vi "MAIN_old.vi"() -> ()   [LabVIEW 2011]
uses:
  <vilib>/userDefined/High Color/IMAQdx.ctl
  <vilib>/vision/driver/NI_Vision_Acquisition_Software.lvlib
panel:
  out "error out 3":errorcluster
  out "error out 2":errorcluster
  out "error out":errorcluster
  out "Image":T1(plugin-control)
  in  "Focused":bool
  out "Ph2 2":dbl
  out "Ph1 2":dbl
  out "[0 255]":dbl
  out "[0 255]":dbl
  in  "Semi2":bool caption="Boolean"
  in  "Semi":bool caption="Boolean"
  out "path":path
  in  "Phase correction 2":bool
  in  "Phase correction":bool caption="Amplitude correction"
  in  "M4":bool
  in  "M4":bool caption="Amplitude correction"
  in  "Hologram:":dbl=1.0
  in  "Hologram:":dbl=1.0
  out "String 2":string
  out "String":string
  out "Ph2":dbl
  in  "Phase:":dbl(slide) scale=0.0..360.0
  out "T2":dbl=100.0
  in  "Tranmitance:":dbl(slide)=100.0 scale=0.0..255.0
  out "Ph1":dbl
  in  "Phase:":dbl(slide) scale=0.0..360.0
  out "T1":dbl=100.0
  in  "Tranmitance:":dbl(slide)=100.0 scale=0.0..255.0
  in  "Parada Total":bool
  in  "Radio Buttons 2":T2(radio)=enum."Radio Selection 6"
  in  "Radio Buttons":T2(radio)=enum."Radio Selection 6"
  in  "Save":bool
  in  "Load Y":bool
  out "selected path 2":path
  in  "Load X":bool
  out "selected path":path
  out "Y position 2":dbl
  in  "Y position 2":dbl(slide)=3.9208633093525176 scale=0.0..10.0
  in  "Fine:":dbl(slide)=5.899280575539568 scale=0.0..10.0
  out "X 2":dbl
  in  "Fine:":dbl(slide)=2.2049689440993787 scale=0.0..10.0
  in  "X position 2":dbl(slide)=1.6770186335403727 scale=0.0..10.0
  out "Y position 1":dbl
  out "X position":dbl
  in  "Fine:":dbl(slide)=0.7636363636363636 scale=0.0..10.0
  in  "Fine:":dbl(slide)=5.590062111801243 scale=0.0..10.0
  in  "X position 1":dbl(slide)=8.409785932721713 scale=0.0..10.0
  in  "Y position":dbl(slide)=2.9454545454545453 scale=0.0..10.0
  out "CGH_x >>":T1(plugin-control)
  out "<< CGH_y":T1(plugin-control)
  # "Arbitrary value settings:"
  # "For gray levels ->"
  # "%"
  # "º"
  # "\\pi rad"
  # "Paraxial"
  # "Arbitrary value settings:"
  # "For gray levels ->"
  # "%"
  # "º"
  # "\\pi rad"
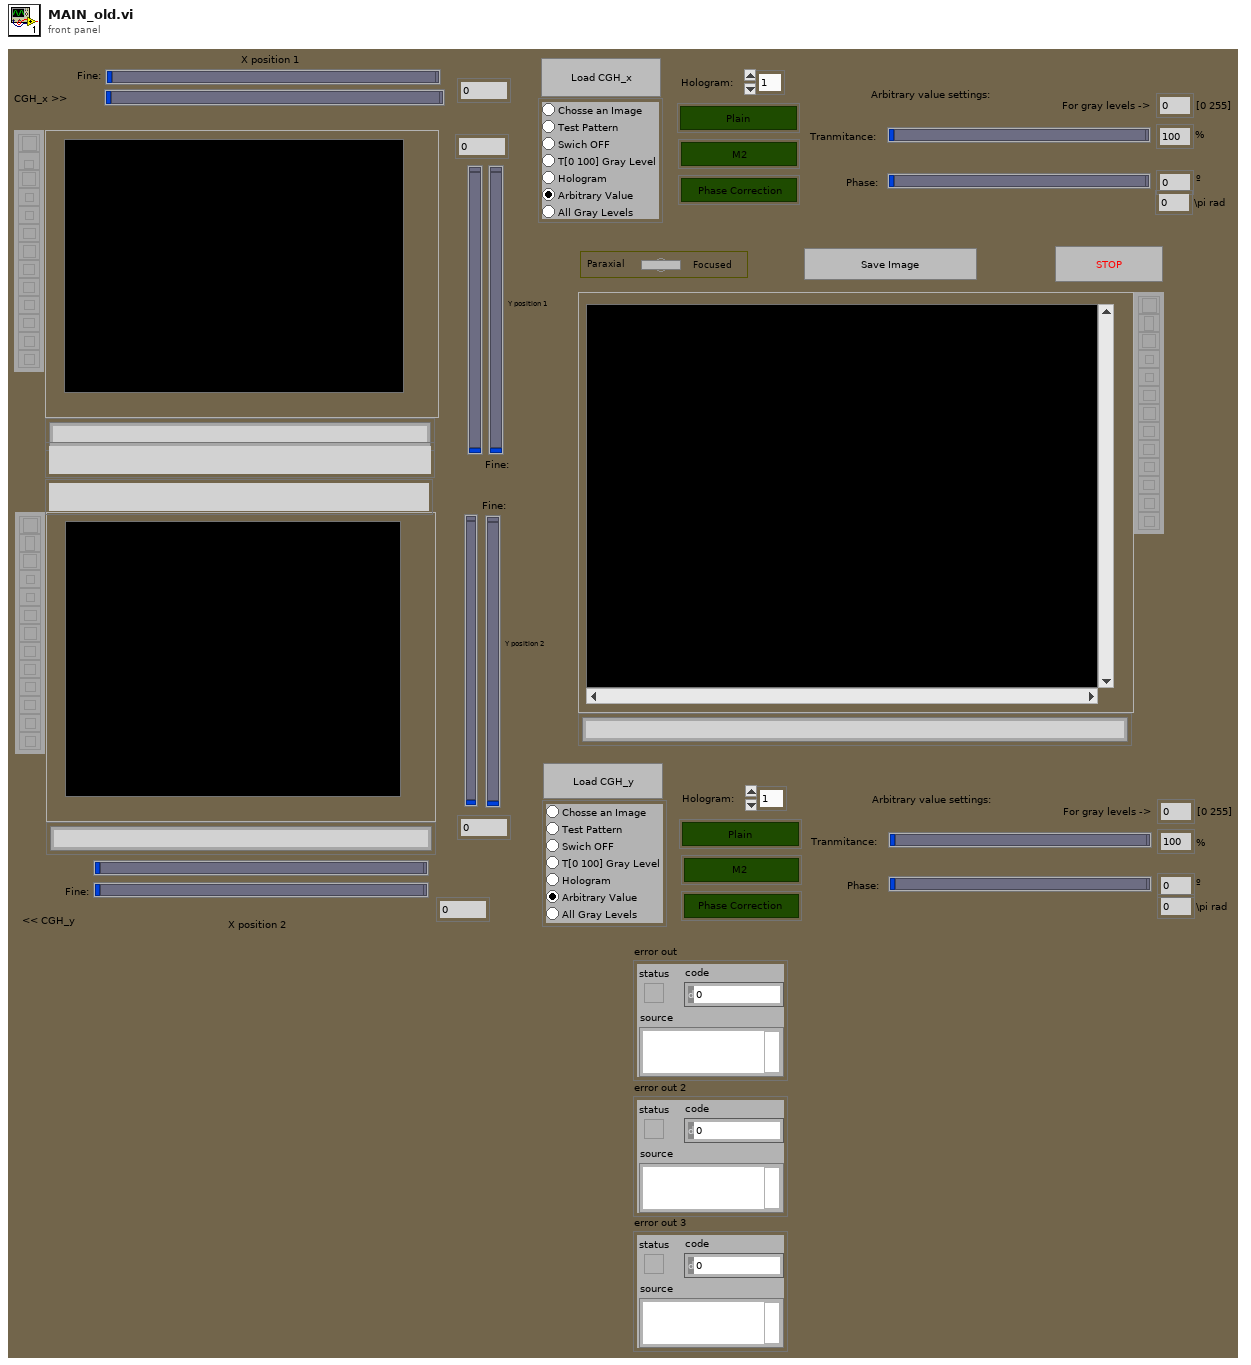
[diagram p1: front panel]
types:
  T1 = typedef "IMAQ Image.ctl" = refnum<image>
  T2 = enum32{"Radio Selection 1", "Radio Selection 2", "Radio Selection 3", "Radio Selection 4", "Radio Selection 5", "Radio Selection 6", "Radio Selection 7"}
  T3 = typedef "IMAQdx.ctl" = refnum<k21>
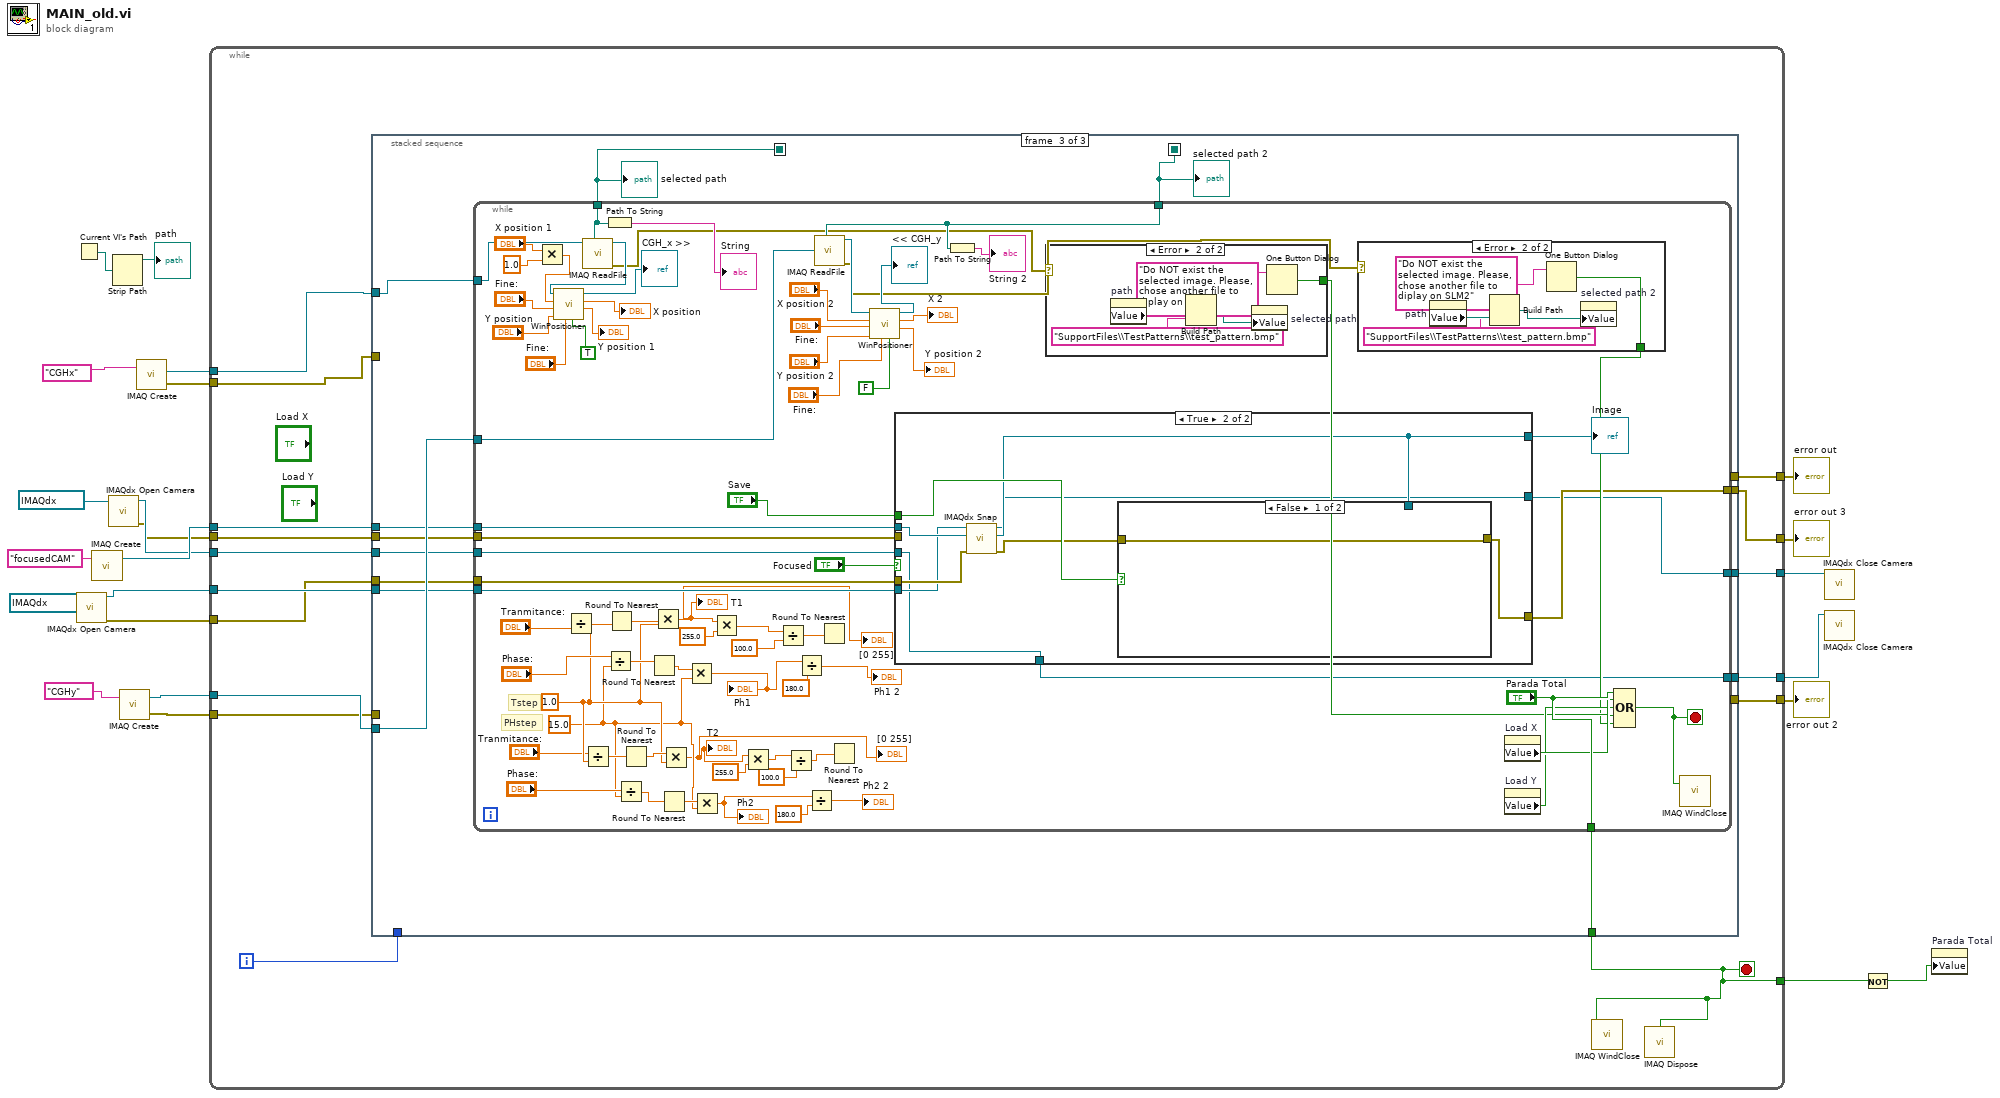
[diagram p0: block diagram]
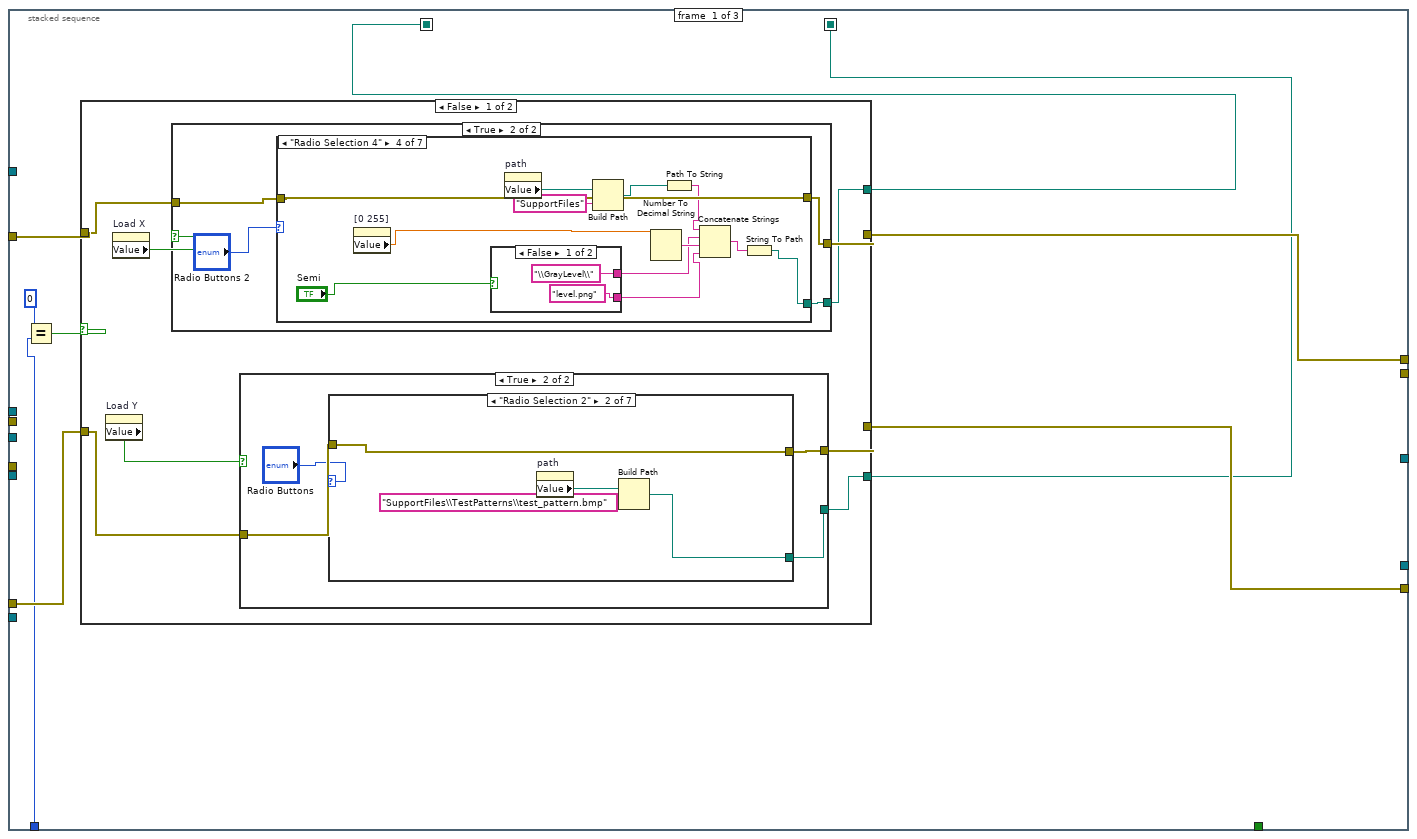
[diagram p2: hidden frame]
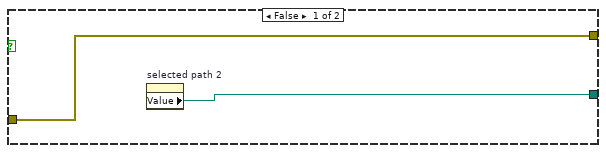
[diagram p3: hidden frame]
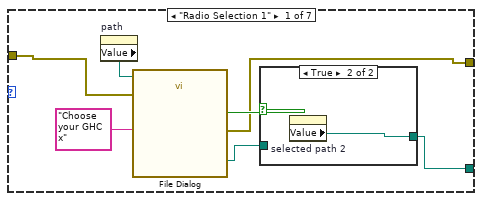
[diagram p4: hidden frame]
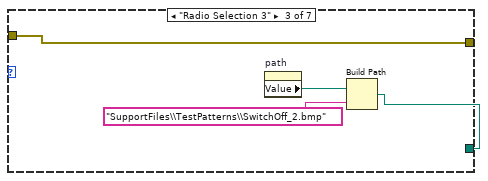
[diagram p6: hidden frame]
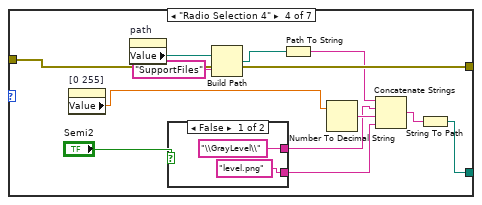
[diagram p7: hidden frame]
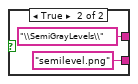
[diagram p8: hidden frame]
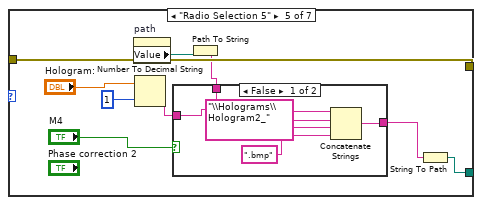
[diagram p9: hidden frame]
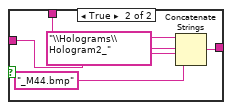
[diagram p10: hidden frame]
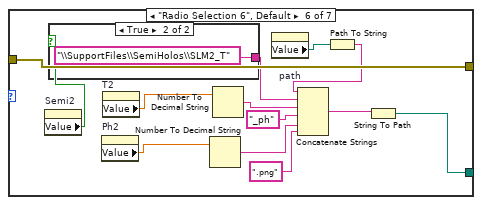
[diagram p11: hidden frame]
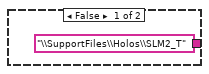
[diagram p12: hidden frame]
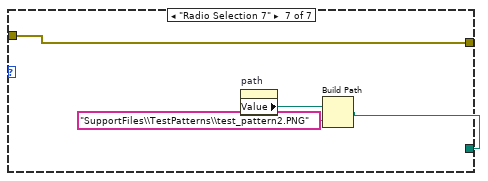
[diagram p13: hidden frame]
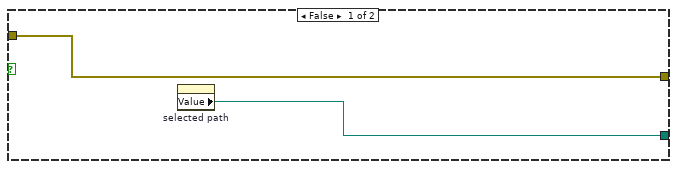
[diagram p14: hidden frame]
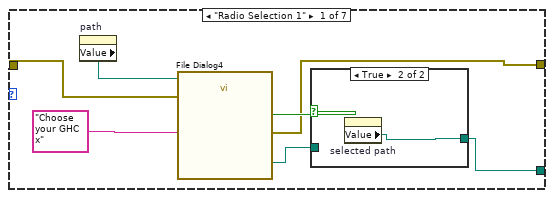
[diagram p15: hidden frame]
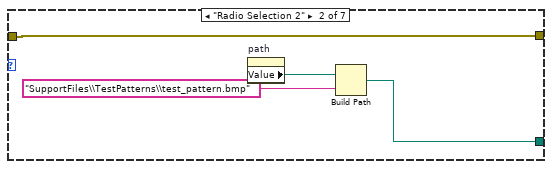
[diagram p17: hidden frame]
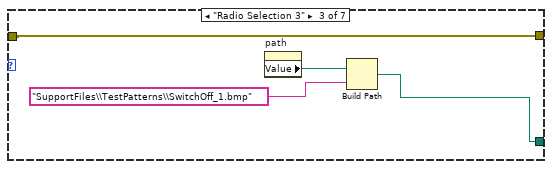
[diagram p18: hidden frame]
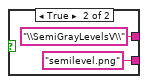
[diagram p19: hidden frame]
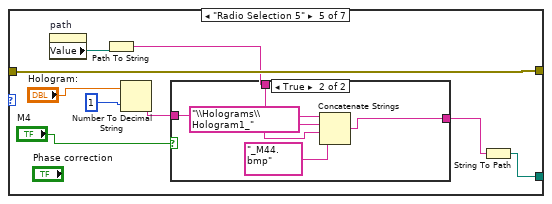
[diagram p20: hidden frame]
diagram:
  n1 = Current VI's Path() -> (path=w16:path)
  n2 = call <vilib>:"IMAQdx Open Camera.vi"("Session In"=T3 "Focused") -> ("error out"=w6:errorcluster, "Session Out"=w7:T3)  [unwired: 9 in]
  n3 = call "IMAQ Create"("Image Name"="focusedCAM") -> ("New Image"=w12:T1)  [unwired: 4 in, 1 out]
  n4 = call <vilib>:"IMAQdx Open Camera.vi"("Session In"=T3 "Paraxial") -> ("error out"=w9:errorcluster, "Session Out"=w10:T3)  [unwired: 9 in]
  n5 = Strip Path(path=w16) -> (stripped path=→"path":path)  [unwired: 1 out]
  n6 = call "IMAQ Create"("Image Name"="CGHy") -> ("New Image"=w20:T1, "error out"=w18:errorcluster)  [unwired: 4 in]
  n7 = call "IMAQ Create"("Image Name"="CGHx") -> ("New Image"=w21:T1, "error out"=w17:errorcluster)  [unwired: 4 in]
  n8 = while {
    tunnel: w21 -> [w39]
    tunnel: w20 -> [w38]
    tunnel: w18 -> [w37]
    tunnel: [w36] -> w4
    tunnel: w17 -> [w35]
    tunnel: [w34] -> w5
    tunnel: [w32] -> w14
    tunnel: w12 -> [w31]
    tunnel: w10 -> [w30]
    tunnel: w9 -> [w29]
    tunnel: w7 -> [w28]
    tunnel: w6 -> [w27]
    tunnel: [w26] -> w3
    tunnel: [w25] -> w2
    tunnel: [w24] -> w1
    i -> [w33]
    stop <- w32 stop-if-true
    n9 = stacked-sequence {
      seq-local: [w40 _ _] -> [_ _ w226]
      seq-local: [w41 _ _] -> [_ _ w225]
      tunnel: w39 -> [_ _ w227]
      tunnel: w38 -> [_ _ w228]
      tunnel: [_ _ w229] -> w32
      tunnel: w37 -> [w48 _ _]
      tunnel: [w47 _ _] -> w36
      tunnel: w35 -> [w46 _ _]
      tunnel: [w45 _ _] -> w34
      tunnel: w33 -> [w44 _ _]
      tunnel: [_ _ w224] -> w26
      tunnel: w31 -> [_ _ w223]
      tunnel: w30 -> [_ _ w222]
      tunnel: w29 -> [_ _ w221]
      tunnel: w28 -> [_ _ w220]
      tunnel: w27 -> [_ _ w219]
      tunnel: [_ _ w218] -> w25
      tunnel: [_ _ w217] -> w24
      frame #0 {
        n10 = Equal?(x=0, y=w44) -> (x = y?=w42:bool)
        n11 = case shown="False" w42 {
          tunnel: [w51 w211] -> w40
          tunnel: [w56 w211] -> w41
          tunnel: w48 -> [w50 w214]
          tunnel: [w53 w214] -> w47
          tunnel: w46 -> [w49 w215]
          tunnel: [w52 w215] -> w45
          frame False {
            n12 = property on="Load Y" class="Bool (strict)"() -> ("Value"=w55:bool)  [unwired: 2 in, 2 out]
            n13 = property on="Load X" class="Bool (strict)"() -> ("Value"=w54:bool)  [unwired: 2 in, 2 out]
            n14 = case shown="True" w54 {
              tunnel: [w135 w138] -> w51
              tunnel: w49 -> [w134 w139]
              tunnel: [w134 w137] -> w52
              frame False {
                n15 = property on="selected path" class="Path"() -> ("Value"=w135:path)  [unwired: 2 in, 2 out]
              }
              frame True {
                n16 = case shown="\"Radio Selection 4\"" "Radio Buttons 2" {
                  tunnel: w139 -> [w142 w152 w156 w168 w181 w204 w210]
                  tunnel: [w141 w149 w153 w165 w179 w198 w207] -> w138
                  tunnel: [w143 w152 w156 w168 w181 w204 w210] -> w137
                  frame "Radio Selection 1" {
                    n17 = property on="path" class="Path"() -> ("Value"=w140:path)  [unwired: 2 in, 2 out]
                    n18 = call "File Dialog4"("start path"=w140, "prompt"="Choose your GHC x", "error in"=w142) -> ("selected path"=w145:path, "cancelled"=w144:bool, "error out"=w143:errorcluster)  [unwired: 9 in, 1 out]
                    n19 = case shown="True" w144 {
                      tunnel: [w147 w148] -> w141
                      tunnel: w145 -> [w147 _]
                      frame False {
                      }
                      frame True {
                        n20 = property on="selected path" class="Path"() -> ("Value"=w148:path)  [unwired: 2 in, 2 out]
                      }
                    }
                  }
                  frame "Radio Selection 2" {
                    n21 = property on="path" class="Path"() -> ("Value"=w151:path)  [unwired: 2 in, 2 out]
                    n22 = Build Path(base path=w151, name or relative path="SupportFiles\\TestPatterns\\test_pattern.bmp") -> (appended path=w149:path)
                  }
                  frame "Radio Selection 3" {
                    n23 = property on="path" class="Path"() -> ("Value"=w155:path)  [unwired: 2 in, 2 out]
                    n24 = Build Path(base path=w155, name or relative path="SupportFiles\\TestPatterns\\SwitchOff_1.bmp") -> (appended path=w153:path)
                  }
                  frame "Radio Selection 4" {
                    n25 = property on="[0 255]" class="DigNum (strict)"() -> ("Value"=w157:dbl)  [unwired: 2 in, 2 out]
                    n26 = case shown="False" "Semi" {
                      tunnel: ["\\GrayLevel\\" ("name or relative path") "\\SemiGrayLevelsV\\" ("name or relative path")] -> w159
                      tunnel: ["level.png" ("string") "semilevel.png" ("string")] -> w158
                      frame False {
                      }
                      frame True {
                      }
                    }
                    n27 = property on="path" class="Path"() -> ("Value"=w164:path)  [unwired: 2 in, 2 out]
                    n28 = Build Path(base path=w164, name or relative path="SupportFiles") -> (appended path=w162:path)
                    n29 = Number To Decimal String(number=w157) -> (decimal integer string=w167:string)  [unwired: 1 in]
                    n30 = Path To String(path=w162) -> (string=w161:string)
                    n31 = Concatenate Strings(w161, w159, w167, w158) -> (w166:string)
                    n32 = String To Path(string=w166) -> (path=w165:path)
                  }
                  frame "Radio Selection 5" {
                    n33 = property on="path" class="Path"() -> ("Value"=w174:path)  [unwired: 2 in, 2 out]
                    n34 = Path To String(path=w174) -> (string=w173:string)
                    n35 = Number To Decimal String(number="Hologram:", width (-)=i16 1) -> (decimal integer string=w177:string)
                    n36 = case shown="True" "M4" {
                      tunnel: [w185 w189] -> w180
                      tunnel: w177 -> [w184 w188]
                      tunnel: w173 -> [w183 w187]
                      frame False {
                        n37 = Concatenate Strings(w183, "\\Holograms\\Hologram1_" ("string"), w184, ".bmp" ("string")) -> (w185:string)
                      }
                      frame True {
                        n38 = Concatenate Strings(w187, "\\Holograms\\Hologram1_" ("string"), w188, "_M44.bmp" ("string")) -> (w189:string)
                      }
                    }
                    n39 = String To Path(string=w180) -> (path=w179:path)
                  }
                  frame "Radio Selection 6", Default {
                    n40 = property on="Semi" class="Bool (strict)"() -> ("Value"=w192:bool)  [unwired: 2 in, 2 out]
                    n41 = case shown="True" w192 {
                      tunnel: ["\\SupportFiles\\Holos\\SLM1_T" ("name or relative path") "\\SupportFiles\\SemiHolos\\SLM1_T" ("name or relative path")] -> w193
                      frame False {
                      }
                      frame True {
                      }
                    }
                    n42 = property on="T1" class="DigNum (strict)"() -> ("Value"=w197:dbl)  [unwired: 2 in, 2 out]
                    n43 = property on="Ph1" class="DigNum (strict)"() -> ("Value"=w196:dbl)  [unwired: 2 in, 2 out]
                    n44 = property on="path" class="Path"() -> ("Value"=w195:path)  [unwired: 2 in, 2 out]
                    n45 = Number To Decimal String(number=w196) -> (decimal integer string=w202:string)  [unwired: 1 in]
                    n46 = Number To Decimal String(number=w197) -> (decimal integer string=w203:string)  [unwired: 1 in]
                    n47 = Path To String(path=w195) -> (string=w194:string)
                    n48 = Concatenate Strings(w194, w193, w203, "_ph" ("Master Thesis (folder)"), w202, ".png" ("Master Thesis (folder)")) -> (w199:string)
                    n49 = String To Path(string=w199) -> (path=w198:path)
                  }
                  frame "Radio Selection 7" {
                    n50 = property on="path" class="Path"() -> ("Value"=w209:path)  [unwired: 2 in, 2 out]
                    n51 = Build Path(base path=w209, name or relative path="SupportFiles\\TestPatterns\\test_pattern2V.PNG") -> (appended path=w207:path)
                  }
                }
              }
            }
            n52 = case shown="True" w55 {
              tunnel: [w58 w61] -> w56
              tunnel: w50 -> [w57 w62]
              tunnel: [w57 w59] -> w53
              frame False {
                n53 = property on="selected path 2" class="Path"() -> ("Value"=w58:path)  [unwired: 2 in, 2 out]
              }
              frame True {
                n54 = case shown="\"Radio Selection 2\"" "Radio Buttons" {
                  tunnel: w62 -> [w65 w75 w79 w91 w104 w127 w133]
                  tunnel: [w64 w72 w76 w88 w102 w121 w130] -> w61
                  tunnel: [w66 w75 w79 w91 w104 w127 w133] -> w59
                  frame "Radio Selection 1" {
                    n55 = property on="path" class="Path"() -> ("Value"=w63:path)  [unwired: 2 in, 2 out]
                    n56 = call "File Dialog"("start path"=w63, "prompt"="Choose your GHC x", "error in"=w65) -> ("selected path"=w68:path, "cancelled"=w67:bool, "error out"=w66:errorcluster)  [unwired: 9 in, 1 out]
                    n57 = case shown="True" w67 {
                      tunnel: [w70 w71] -> w64
                      tunnel: w68 -> [w70 _]
                      frame False {
                      }
                      frame True {
                        n58 = property on="selected path 2" class="Path"() -> ("Value"=w71:path)  [unwired: 2 in, 2 out]
                      }
                    }
                  }
                  frame "Radio Selection 2" {
                    n59 = property on="path" class="Path"() -> ("Value"=w74:path)  [unwired: 2 in, 2 out]
                    n60 = Build Path(base path=w74, name or relative path="SupportFiles\\TestPatterns\\test_pattern.bmp") -> (appended path=w72:path)
                  }
                  frame "Radio Selection 3" {
                    n61 = property on="path" class="Path"() -> ("Value"=w78:path)  [unwired: 2 in, 2 out]
                    n62 = Build Path(base path=w78, name or relative path="SupportFiles\\TestPatterns\\SwitchOff_2.bmp") -> (appended path=w76:path)
                  }
                  frame "Radio Selection 4" {
                    n63 = property on="[0 255]" class="DigNum (strict)"() -> ("Value"=w80:dbl)  [unwired: 2 in, 2 out]
                    n64 = property on="path" class="Path"() -> ("Value"=w87:path)  [unwired: 2 in, 2 out]
                    n65 = case shown="False" "Semi2" {
                      tunnel: ["\\GrayLevel\\" ("name or relative path") "\\SemiGrayLevels\\" ("name or relative path")] -> w83
                      tunnel: ["level.png" ("string") "semilevel.png" ("string")] -> w82
                      frame False {
                      }
                      frame True {
                      }
                    }
                    n66 = Build Path(base path=w87, name or relative path="SupportFiles") -> (appended path=w85:path)
                    n67 = Path To String(path=w85) -> (string=w84:string)
                    n68 = Number To Decimal String(number=w80) -> (decimal integer string=w90:string)  [unwired: 1 in]
                    n69 = Concatenate Strings(w84, w83, w90, w82) -> (w89:string)
                    n70 = String To Path(string=w89) -> (path=w88:path)
                  }
                  frame "Radio Selection 5" {
                    n71 = property on="path" class="Path"() -> ("Value"=w97:path)  [unwired: 2 in, 2 out]
                    n72 = Number To Decimal String(number="Hologram:", width (-)=i16 1) -> (decimal integer string=w98:string)
                    n73 = Path To String(path=w97) -> (string=w96:string)
                    n74 = case shown="False" "M4" {
                      tunnel: w96 -> [w107 w114]
                      tunnel: [w105 w111] -> w103
                      tunnel: w98 -> [w108 w112]
                      frame False {
                        n75 = Concatenate Strings(w107, "\\Holograms\\Hologram2_" ("string"), w108, ".bmp" ("string")) -> (w105:string)
                      }
                      frame True {
                        n76 = Concatenate Strings(w114, "\\Holograms\\Hologram2_" ("string"), w112, "_M44.bmp" ("string")) -> (w111:string)
                      }
                    }
                    n77 = String To Path(string=w103) -> (path=w102:path)
                  }
                  frame "Radio Selection 6", Default {
                    n78 = property on="Semi2" class="Bool (strict)"() -> ("Value"=w118:bool)  [unwired: 2 in, 2 out]
                    n79 = case shown="True" w118 {
                      tunnel: ["\\SupportFiles\\Holos\\SLM2_T" ("name or relative path") "\\SupportFiles\\SemiHolos\\SLM2_T" ("name or relative path")] -> w115
                      frame False {
                      }
                      frame True {
                      }
                    }
                    n80 = property on="Ph2" class="DigNum (strict)"() -> ("Value"=w119:dbl)  [unwired: 2 in, 2 out]
                    n81 = property on="T2" class="DigNum (strict)"() -> ("Value"=w120:dbl)  [unwired: 2 in, 2 out]
                    n82 = Number To Decimal String(number=w119) -> (decimal integer string=w125:string)  [unwired: 1 in]
                    n83 = Number To Decimal String(number=w120) -> (decimal integer string=w126:string)  [unwired: 1 in]
                    n84 = property on="path" class="Path"() -> ("Value"=w117:path)  [unwired: 2 in, 2 out]
                    n85 = Path To String(path=w117) -> (string=w116:string)
                    n86 = Concatenate Strings(w116, w115, w126, "_ph" ("Master Thesis (folder)"), w125, ".png" ("Master Thesis (folder)")) -> (w122:string)
                    n87 = String To Path(string=w122) -> (path=w121:path)
                  }
                  frame "Radio Selection 7" {
                    n88 = property on="path" class="Path"() -> ("Value"=w132:path)  [unwired: 2 in, 2 out]
                    n89 = Build Path(base path=w132, name or relative path="SupportFiles\\TestPatterns\\test_pattern2.PNG") -> (appended path=w130:path)
                  }
                }
              }
            }
          }
          frame True {
            n90 = property on="path" class="Path"() -> ("Value"=w213:path)  [unwired: 2 in, 2 out]
            n91 = Build Path(base path=w213, name or relative path="SupportFiles\\TestPatterns\\test_pattern.bmp") -> (appended path=w211:path)
          }
        }
      }
      frame #1 {
        w216 = FALSE ("Load X")
        n92 = property on="Radio Selection 6" class="Bool (strict)" props=["Value"]() -> ()  [unwired: 2 in, 3 out]
        n93 = property on="Radio Selection 6" class="Bool (strict)" props=["Value"]() -> ()  [unwired: 2 in, 3 out]
        n94 = property on="Load X" class="Bool (strict)"("Value"=w216) -> ()  [unwired: 2 in, 2 out]
        n95 = property on="Load Y" class="Bool (strict)"("Value"=w216) -> ()  [unwired: 2 in, 2 out]
      }
      frame #2 {
        n96 = while {
          tunnel: ["Parada Total"] -> w229
          tunnel: w226 -> [w284]
          tunnel: w225 -> [w272]
          tunnel: w228 -> [w303]
          tunnel: w227 -> [w302]
          tunnel: [w243] -> w224
          tunnel: w223 -> [w239]
          tunnel: w222 -> [w238]
          tunnel: w221 -> [w237]
          tunnel: w220 -> [w236]
          tunnel: w219 -> [w235]
          tunnel: [w234] -> w218
          tunnel: [w233] -> w217
          stop <- w249 stop-if-true
          w253 = 15.0 ("x")
          w262 = 1.0 ("x")
          # "PHstep"
          # "Tstep"
          n97 = Multiply(x="X position 1", y=1.0 ("x")) -> (x*y=w288:dbl)
          n98 = Divide(x="Tranmitance:", y=w262) -> (x/y=w270:dbl)
          n99 = call "IMAQ ReadFile"("File Path"=w284, "Image"=w302) -> ("error out"=w271:errorcluster, "Image Out"=w291:T1)  [unwired: 5 in, 3 out]
          n100 = call "WinPositioner.vi"("Image"=w291, "X position"=w288, "Fine X position"="Fine:", "Y position"="Y position", "Fine Y position"="Fine:", "Display?"=TRUE) -> ("CGH_x"=→"CGH_x >>":T1, "X position"=→"X position":dbl, "Y position"=→"Y position 1":dbl)  [unwired: 2 in]
          n101 = Divide(x="Tranmitance:", y=w262) -> (x/y=w264:dbl)
          n102 = Path To String(path=w284) -> (string=→"String":string)
          n103 = Divide(x="Phase:", y=w253) -> (x/y=w300:dbl)
          n104 = Round To Nearest(number=w270) -> (nearest integer value=w297:dbl)
          n105 = Divide(x="Phase:", y=w253) -> (x/y=w255:dbl)
          n106 = Round To Nearest(number=w264) -> (nearest integer value=w263:dbl)
          n107 = Round To Nearest(number=w300) -> (nearest integer value=w298:dbl)
          n108 = Multiply(x=w297, y=w262) -> (x*y=w230:dbl)
          "T1" <- w230
          "[0 255]" <- w230
          n109 = Round To Nearest(number=w255) -> (nearest integer value=w254:dbl)
          n110 = Multiply(x=w263, y=w262) -> (x*y=w231:dbl)
          "T2" <- w231
          "[0 255]" <- w231
          n111 = Multiply(x=w298, y=w253) -> (x*y=w265:dbl)
          "Ph1" <- w265
          n112 = Multiply(x=w254, y=w253) -> (x*y=w252:dbl)
          "Ph2" <- w252
          n113 = Multiply(x=w230, y=255.0) -> (x*y=w268:dbl)
          n114 = Multiply(x=w231, y=255.0) -> (x*y=w260:dbl)
          n115 = Divide(x=w268, y=100.0) -> (x/y=w266:dbl)
          n116 = Divide(x=w260, y=100.0) -> (x/y=w258:dbl)
          n117 = Divide(x=w265, y=180.0) -> (x/y=→"Ph1 2":dbl)
          n118 = Divide(x=w252, y=180.0) -> (x/y=→"Ph2 2":dbl)
          n119 = call "IMAQ ReadFile"("File Path"=w272, "Image"=w303) -> ("error out"=w240:errorcluster, "Image Out"=w274:T1)  [unwired: 5 in, 3 out]
          n120 = Round To Nearest(number=w266) -> ()  [unwired: 1 out]
          n121 = Round To Nearest(number=w258) -> ()  [unwired: 1 out]
          n122 = call "WinPositioner.vi"("Image"=w274, "X position"="X position 2", "Fine X position"="Fine:", "Y position"="Y position 2", "Fine Y position"="Fine:", "Display?"=FALSE) -> ("CGH_x"=→"<< CGH_y":T1, "X position"=→"X 2":dbl, "Y position"=→"Y position 2":dbl)  [unwired: 2 in]
          n123 = case shown="True" "Focused" {
            tunnel: "Save" -> [w312 w334]
            tunnel: [w313 w335] -> w243
            tunnel: [w311 w332] -> w241
            tunnel: w239 -> [w307 w333]
            tunnel: w238 -> [w310 w327]
            tunnel: w237 -> [w309 _]
            tunnel: w236 -> [w305 w329]
            tunnel: w235 -> [_ w331]
            tunnel: [w305 w328] -> w234
            tunnel: [w306 w327] -> w233
            frame False {
              n124 = call <vilib>:"IMAQdx Snap.vi"("error in"=w309, "Image In"=w307, "Session In"=w310) -> ("error out"=w308:errorcluster, "Image Out"=w311:T1, "Session Out"=w306:T3)  [unwired: 6 in]
              n125 = case shown="False" w312 {
                tunnel: [w314 w317] -> w313
                tunnel: w311 -> [_ w316]
                tunnel: w308 -> [w314 w315]
                frame False {
                }
                frame True {
                  n126 = property on="path" class="Path"() -> ("Value"=w325:path)  [unwired: 2 in, 2 out]
                  n127 = Build Path(base path=w325, name or relative path="Images") -> (appended path=w324:path)
                  n128 = call "File Dialog3"("start path"=w324, "prompt"="Save image", "button label"="Save", "error in"=w315, "pattern (all files)"=".png", "pattern label"="PNG") -> ("selected path"=w326:path, "error out"=w318:errorcluster)  [unwired: 6 in, 2 out]
                  n129 = call-poly "IMAQ Write File 2"("error in (no error)"=w318, "File Path"=w326, "Image"=w316) -> ("error out"=w317:errorcluster)  [unwired: 7 in, 1 out]
                }
              }
            }
            frame True {
              n130 = call <vilib>:"IMAQdx Snap.vi"("error in"=w331, "Image In"=w333, "Session In"=w329) -> ("error out"=w330:errorcluster, "Image Out"=w332:T1, "Session Out"=w328:T3)  [unwired: 6 in]
              n131 = case shown="False" w334 {
                tunnel: [w336 w346] -> w335
                tunnel: w332 -> [_ w338]
                tunnel: w330 -> [w336 w337]
                frame False {
                }
                frame True {
                  n132 = property on="path" class="Path"() -> ("Value"=w345:path)  [unwired: 2 in, 2 out]
                  n133 = Build Path(base path=w345, name or relative path="Images") -> (appended path=w344:path)
                  n134 = call "File Dialog2"("start path"=w344, "prompt"="Save image", "button label"="Save", "error in"=w337, "pattern (all files)"=".png", "pattern label"="PNG") -> ("selected path"=w348:path, "error out"=w347:errorcluster)  [unwired: 6 in, 2 out]
                  n135 = call-poly "IMAQ Write File 2"("error in (no error)"=w347, "File Path"=w348, "Image"=w338) -> ("error out"=w346:errorcluster)  [unwired: 7 in, 1 out]
                }
              }
            }
          }
          "Image" <- w241
          n136 = Path To String(path=w272) -> (string=→"String 2":string)
          n137 = case shown="Error" w271 {
            tunnel: [FALSE ("true") w357] -> w245
            frame No Error {
            }
            frame Error {
              n138 = property on="path" class="Path"() -> ("Value"=w359:path)  [unwired: 2 in, 2 out]
              n139 = Build Path(base path=w359, name or relative path="SupportFiles\\TestPatterns\\test_pattern.bmp") -> (appended path=w358:path)
              n140 = property on="selected path" class="Path"("Value"=w358) -> ()  [unwired: 2 in, 2 out]
              n141 = One Button Dialog(message="Do NOT exist the selected image. Please, chose another file to diplay on SLM1") -> (true=w357:bool)  [unwired: 1 in]
            }
          }
          n142 = case shown="Error" w240 {
            tunnel: [FALSE ("true") w352] -> w244
            frame No Error {
            }
            frame Error {
              n143 = property on="path" class="Path"() -> ("Value"=w354:path)  [unwired: 2 in, 2 out]
              n144 = Build Path(base path=w354, name or relative path="SupportFiles\\TestPatterns\\test_pattern.bmp") -> (appended path=w353:path)
              n145 = One Button Dialog(message="Do NOT exist the selected image. Please, chose another file to diplay on SLM2") -> (true=w352:bool)  [unwired: 1 in]
              n146 = property on="selected path 2" class="Path"("Value"=w353) -> ()  [unwired: 2 in, 2 out]
            }
          }
          n147 = property on="Load X" class="Bool (strict)"() -> ("Value"=w247:bool)  [unwired: 2 in, 2 out]
          n148 = property on="Load Y" class="Bool (strict)"() -> ("Value"=w246:bool)  [unwired: 2 in, 2 out]
          n149 = Compound Arithmetic op=OR("Parada Total", w247, w246, w245, w244) -> (w249:bool)
          n150 = call "IMAQ WindClose"("Close All Windows (False)"=w249) -> ()  [unwired: 5 in, 1 out]
        }
        "selected path" <- w226
        "selected path 2" <- w225
      }
    }
    n151 = call "IMAQ WindClose"("Close All Windows (False)"=w32) -> ()  [unwired: 5 in, 1 out]
    n152 = call "IMAQ Dispose"("All Images? (No)"=w32) -> ()  [unwired: 5 in, 1 out]
  }
  "error out" <- w5
  "error out 2" <- w4
  "error out 3" <- w3
  n153 = call <vilib>:"IMAQdx Close Camera.vi"("Session In"=w2) -> ()  [unwired: 10 in, 1 out]
  n154 = call <vilib>:"IMAQdx Close Camera.vi"("Session In"=w1) -> ()  [unwired: 10 in, 1 out]
  n155 = Not(x=w14) -> (.not. x?=w19:bool)
  n156 = property on="Parada Total" class="Bool (strict)"("Value"=w19) -> ()  [unwired: 2 in, 2 out]
